vi "Read System Status For No response.vi"(6 "error in":errorcluster, 8 "MaxRead":i32, 9 "Channel in":u16) -> (0 "error out":errorcluster, 1 "Messages":T2(array[cluster]), 2 "Pass":bool, 3 "Channel out":u16)   [LabVIEW 2023]
uses:
  7e6a34f5-6666-41a7-b638-f367e94293a1.vi
  Communication/PCAN2023/PCAN API.lvlib
panel:
  out "MessageBuffer out 3":T1 {"ID" format="%.0x"; "DATA[0]" format="%.0x"; "DATA[1]" format="%.0x"; "DATA[2]" format="%.0x"; "DATA[3]" format="%.0x"; "DATA[4]" format="%.0x"; "DATA[5]" format="%.0x"; "DATA[6]" format="%.0x"; "DATA[7]" format="%.0x"}
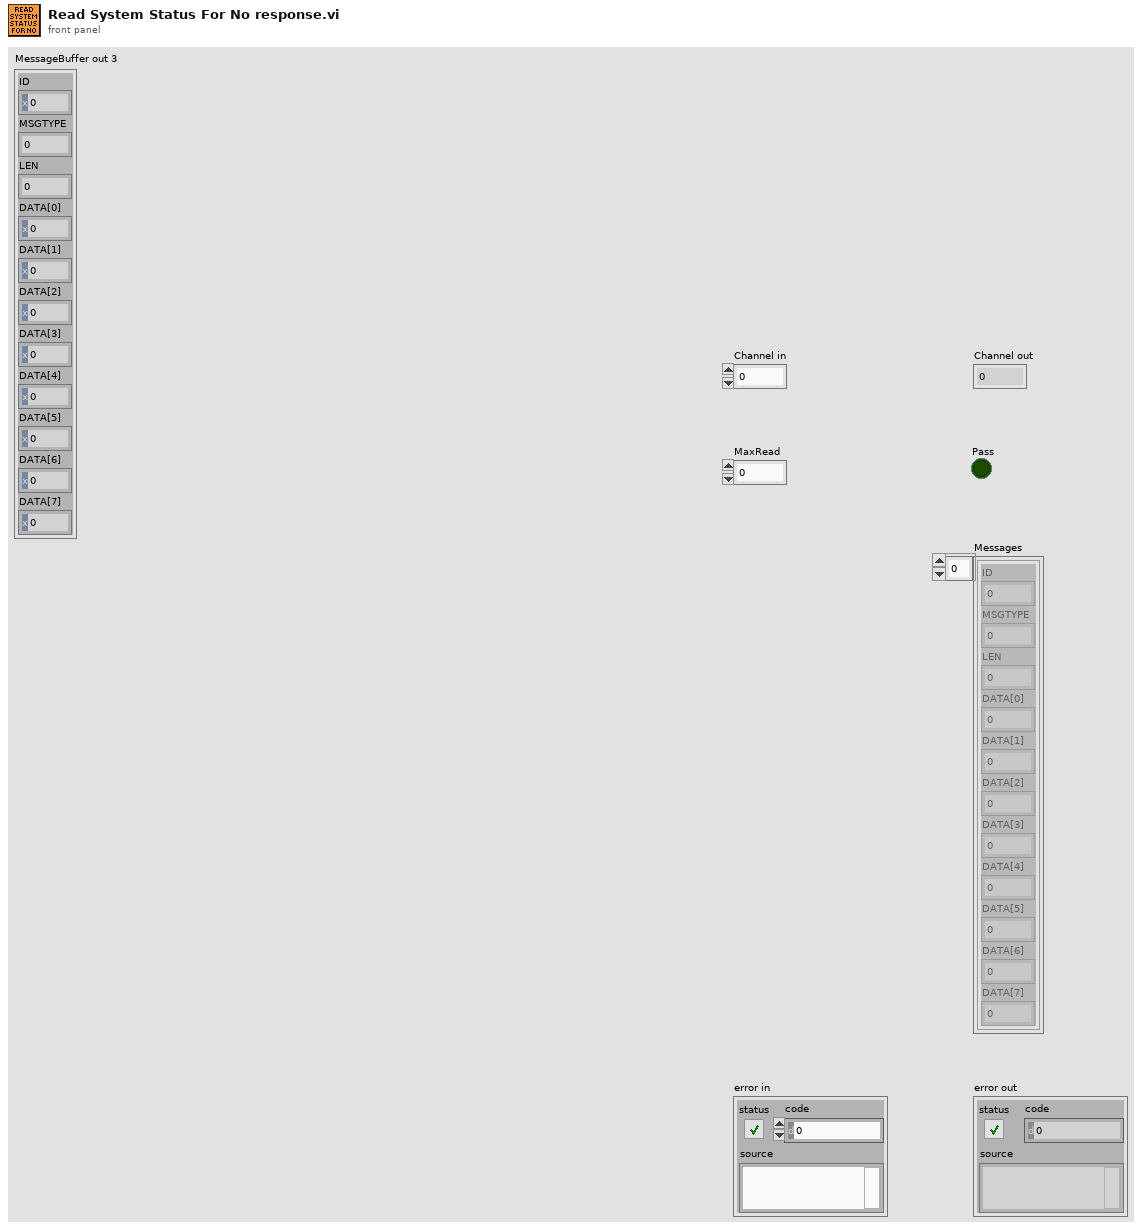
[diagram p1: front panel]
types:
  T1 = cluster{"ID":u32, "MSGTYPE":u8, "LEN":u8, "DATA[0]":u8, "DATA[1]":u8, "DATA[2]":u8, "DATA[3]":u8, "DATA[4]":u8, "DATA[5]":u8, "DATA[6]":u8, "DATA[7]":u8}
  T2 = cluster{"ID":u32, "MSGTYPE":u8, "LEN":u8, "DATA[0]":u8, "DATA[1]":u8, "DATA[2]":u8, "DATA[3]":u8, "DATA[4]":u8, "DATA[5]":u8, "DATA[6]":u8, "DATA[7]":u8}[]
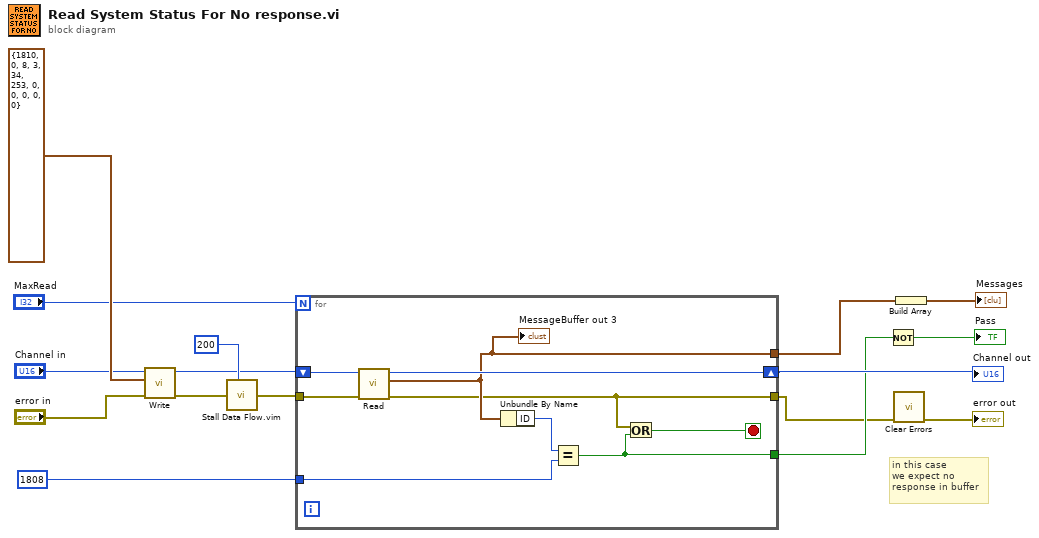
[diagram p0: block diagram]
diagram:
  # "in this case\nwe expect no \nresponse in buffer"
  n1 = call "Write.vi"("error in"="error in", "MessageBuffer"=T1 {"ID"=1810, "MSGTYPE"=0, "LEN"=8, "DATA[0]"=3, "DATA[1]"=34, "DATA[2]"=253, "DATA[3]"=0, "DATA[4]"=0, "DATA[5]"=0, "DATA[6]"=0, "DATA[7]"=0}, "Channel"="Channel in") -> ("error out"=w15:errorcluster, "Channel out"=w9:u16)  [unwired: 5 in, 2 out]
  n2 = call "Stall Data Flow.vim"("value in"=w15, "milliseconds to wait"=u32 200) -> ("value out"=w8:errorcluster)  [unwired: 1 out]
  n3 = for {
    N: "MaxRead" -> [_]
    shift-right: [w24] -> w5
    shift-left: w9 -> [w25]
    tunnel: u32 1808 ("ID") -> [w22]
    tunnel: [w20] -> w4
    tunnel: w8 -> [w21]
    tunnel: [w19] -> w2
    tunnel: [w17] -> w3
    stop <- w18 stop-if-true
    n4 = call "Read.vi"("error in"=w21, "Channel"=w25) -> ("error out"=w19:errorcluster, "MessageBuffer out"=w20:T1, "Channel out"=w24:u16)  [unwired: 6 in, 1 out]
    "MessageBuffer out 3" <- w20
    n5 = Unbundle By Name(w20) -> ("ID"=w23:u32)
    n6 = Equal?(x=w23, y=w22) -> (x = y?=w17:bool)
    n7 = Or(x=w19, y=w17) -> (x .or. y?=w18:bool)
  }
  "Channel out" <- w5
  n8 = Not(x=w3) -> (.not. x?=→"Pass":bool)
  n9 = call <vilib>:"Clear Errors.vi"("error in (no error)"=w2) -> ("error out"=→"error out":errorcluster)  [unwired: 5 in, 1 out]
  n10 = Build Array(w4) -> (→"Messages":T2)
